vi "Projet01.vi"() -> ()   [LabVIEW 2016]
uses:
  <vilib>/Analysis/3filter.llb/Filter Passband Type.ctl
  <vilib>/Utility/file.llb/Read Delimited Spreadsheet (DBL).vi
  <vilib>/Utility/file.llb/Read Delimited Spreadsheet (string).vi
  <vilib>/Analysis/3filter.llb/Chebyshev Filter (DBL).vi
  <vilib>/Analysis/NI_AALBase.lvlib
panel:
  out "Total Samples":dbl
  out "Median":dbl
  out "Maximum":dbl
  out "Mode":dbl
  out "Variance":dbl
  in  "sampling freq: fs":dbl=1.0 format="%0.2f"
  in  "high cutoff freq: fh":dbl=0.45000000000000007 format="%0.2f"
  in  "low cutoff freq: fl":dbl=0.125 format="%0.4f"
  in  "filter type":T1
  in  "order":i32=2
  out "Signal filtré":T2
  out "signal":dynamicdata(graph)
  out "Signal avec bruit":dynamicdata(graph)
  in  "Noise amplitude":dbl=0.6
  out "all rows 2":string[][](array[string])
  out "all rows":dbl[][](array[numeric])
  in  "file path (dialog if empty)":path
  # "Recuperation des données"
  # "Statistiques"
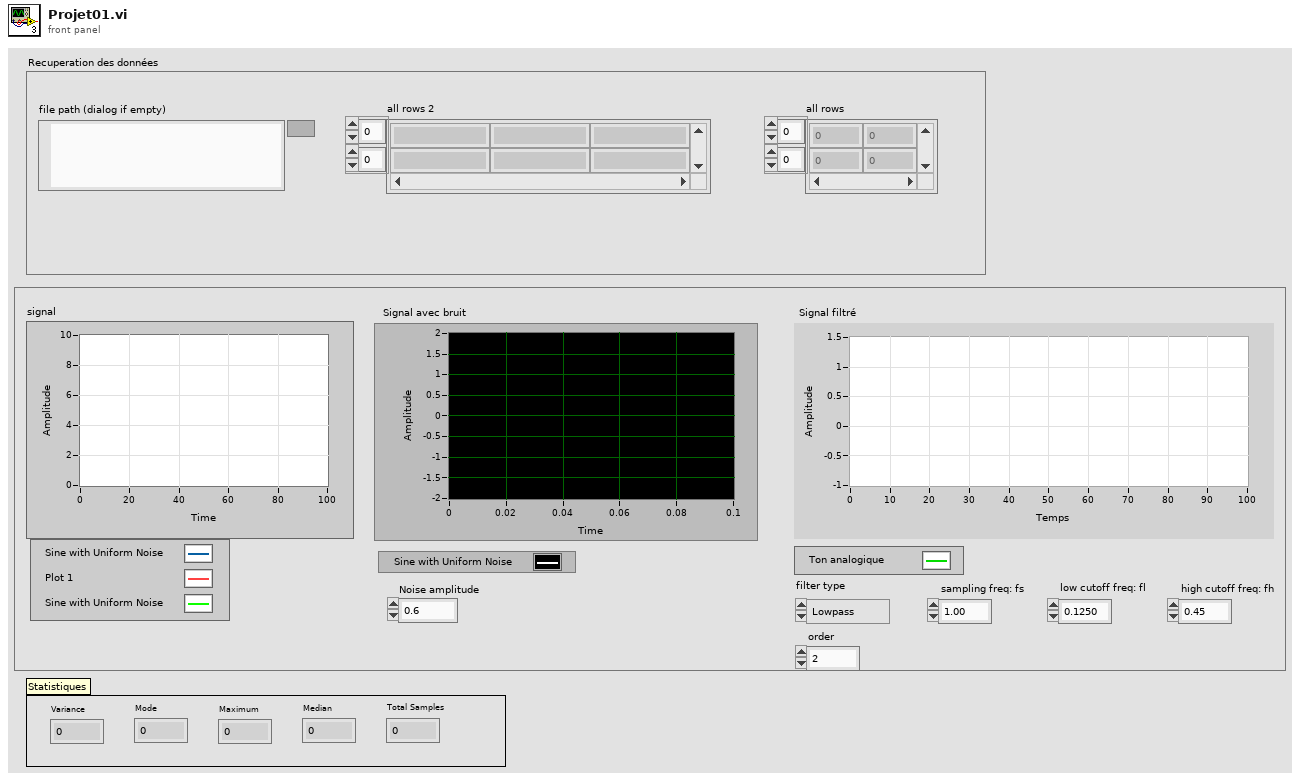
[diagram p1: front panel]
types:
  T1 = typedef "NI_AALBase.lvlib/Filter Passband Type.ctl" = enum32{"Lowpass", "Highpass", "Bandpass", "Bandstop"}
  T2 = typedef "Projet-traitement-de-signal1" = dbl[]
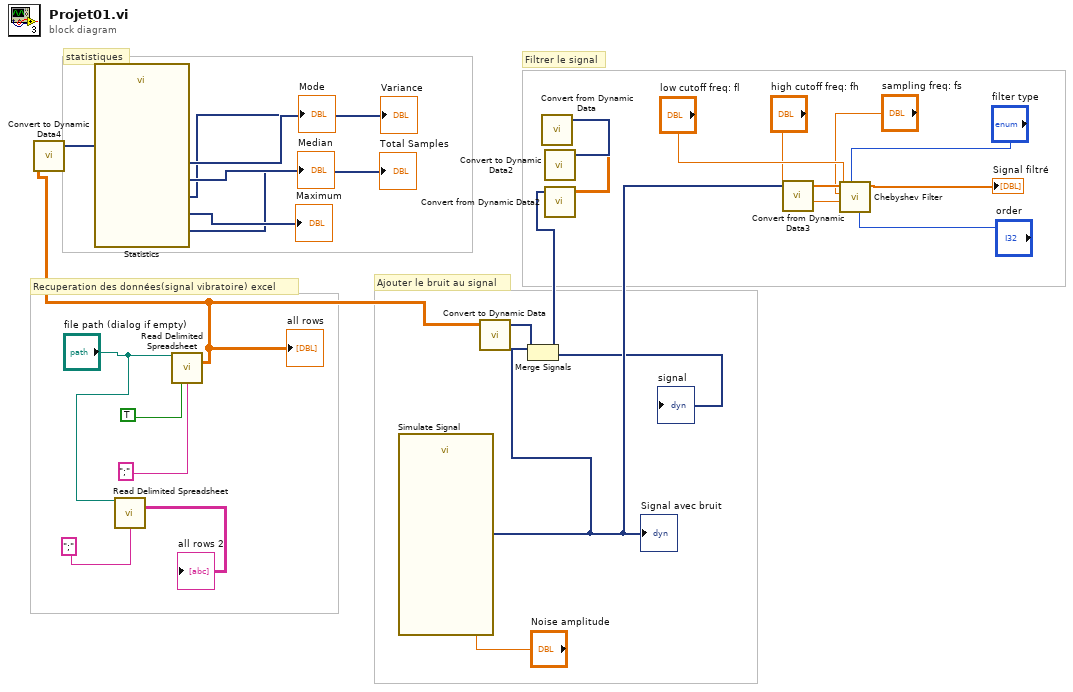
[diagram p0: block diagram]
diagram:
  # "Filtrer le signal"
  # "Ajouter le bruit au signal"
  # "Recuperation des données(signal vibratoire) excel"
  # "statistiques"
  n1 = call-poly <vilib>:"Read Delimited Spreadsheet.vi"("file path (dialog if empty)"="file path (dialog if empty)", "delimiter (\\t)"=";" ("delimiter (\\t)")) -> ("all rows"=→"all rows 2":string[][])  [unwired: 8 in, 5 out]
  n2 = call-poly <vilib>:"Read Delimited Spreadsheet.vi"("file path (dialog if empty)"="file path (dialog if empty)", "transpose? (F)"=TRUE, "delimiter (\\t)"=";" ("delimiter (\\t)")) -> ("all rows"=w8:dbl[][])  [unwired: 7 in, 5 out]
  "all rows" <- w8
  n3 = call "Convert to Dynamic Data4"("2D Array"=w8) -> ("Dynamic Data Type"=w7:dynamicdata)  [unwired: 3 in]
  n4 = call "Statistics"("Signals"=w7) -> ("Total Samples"=→"Total Samples":dynamicdata, "Mode"=→"Mode":dynamicdata, "Median"=→"Median":dynamicdata, "Variance"=→"Variance":dynamicdata, "Maximum"=→"Maximum":dynamicdata)  [unwired: 21 in, 1 out]
  n5 = call "Simulate Signal"("Noise amplitude"="Noise amplitude") -> ("Sine with Uniform Noise"=w16:dynamicdata)  [unwired: 13 in, 1 out]
  "Signal avec bruit" <- w16
  n6 = call "Convert to Dynamic Data"("2D Array"=w8) -> ("Dynamic Data Type"=w19:dynamicdata)  [unwired: 3 in]
  n7 = Merge Signals(w16, w19) -> (w1:dynamicdata)
  "signal" <- w1
  n8 = call "Convert from Dynamic Data2"("Dynamic Data Type"=w1) -> ("Array"=w17:dbl[][])  [unwired: 3 in]
  n9 = call "Convert to Dynamic Data2"("2D Array"=w17) -> ("Dynamic Data Type"=w18:dynamicdata)  [unwired: 3 in]
  n10 = call "Convert from Dynamic Data"("Dynamic Data Type"=w18) -> ()  [unwired: 3 in, 1 out]
  n11 = call "Convert from Dynamic Data3"("Dynamic Data Type"=w16) -> ("Array"=w15:dbl[])  [unwired: 3 in]
  n12 = call-poly <vilib>:"Chebyshev Filter.vi"("order"="order", "filter type"="filter type", "low cutoff freq: fl"="low cutoff freq: fl", "high cutoff freq: fh"="high cutoff freq: fh", "sampling freq: fs"="sampling freq: fs", "X"=w15) -> ("Filtered X"=→"Signal filtré":dbl[])  [unwired: 4 in, 1 out]
